vi "Algo prédictif.vi"(11 "Puissance intan.":dbl) -> (3 "Puissance prédite":dbl)   [LabVIEW 2018]
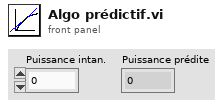
[diagram p1: front panel]
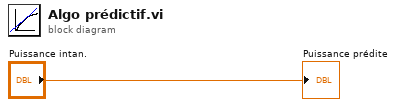
[diagram p0: block diagram]
diagram:
  "Puissance prédite" <- "Puissance intan."
